vi "Test_Toolbar-Global.vi"() -> ()   [LabVIEW 2020, in "Sgraph_lib_V1.lvlib"]
uses:
  Builds/Sgraph_lib_V1.lvlib
  <vilib>/Utility/miscctls.llb/LVPoint32TypeDef.ctl
panel:
  in  "Coords":T1
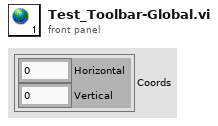
[diagram p1: front panel]
types:
  T1 = typedef "LVPoint32TypeDef.ctl" = cluster{"Horizontal":i32, "Vertical":i32}
diagram:
